vi "niDTS Comm String Initialize.vi"(0 "Session Name ()":string, 5 "Plugin Path":path, 7 "Logger":T2, 11 "error in (no error)":errorcluster) -> (4 "Comm String Handle":T1, 15 "error out":errorcluster)   [LabVIEW 2015, in "niDTS CommLib.lvlib"]
uses:
  niDTS CommLib.lvlib
  Framework/Logger/Includes/niDTS Logger INC Handle.ctl
  Framework/Logger/Objects/BASE_class/niDTS Logger.lvclass
  Includes/niDTS Comm String INC Handle.ctl
  Objects/String_class/niDTS Comm String.lvclass
  Framework/Session/Objects/BASE_class/niDTS Session.lvclass
  Framework/niDTS Framework.lvlib
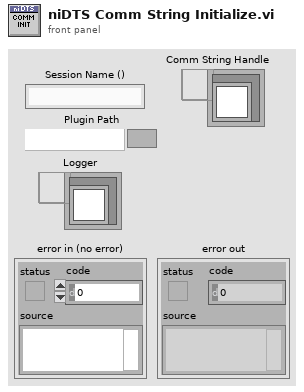
[diagram p1: front panel]
types:
  T1 = typedef "niDTS CommLib.lvlib/niDTS Comm String INC Handle.ctl" = refnum<data-value>
  T2 = typedef "niDTS Framework.lvlib/niDTS Logger INC Handle.ctl" = refnum<data-value>
  T3 = typedef "niDTS Framework.lvlib/niDTS Session INC Handle.ctl" = refnum<data-value>
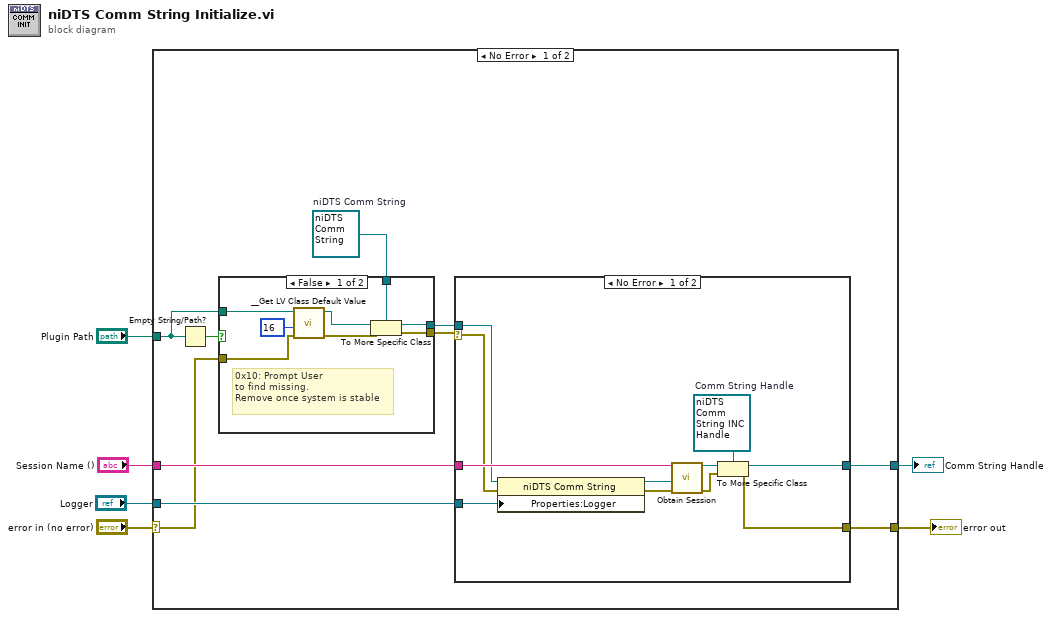
[diagram p0: block diagram]
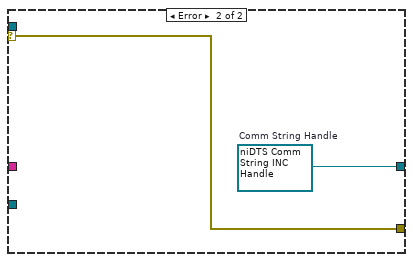
[diagram p2: hidden frame]
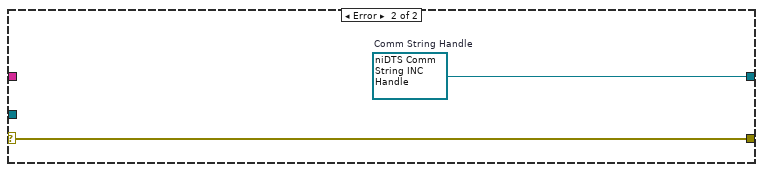
[diagram p4: hidden frame]
diagram:
  n1 = case shown="No Error" "error in (no error)" {
    selector: "error in (no error)" -> [w10 w41]
    tunnel: "Session Name ()" -> [w16 _]
    tunnel: [w15 w41] -> w5
    tunnel: "Logger" -> [w14 _]
    tunnel: "Plugin Path" -> [w11 _]
    tunnel: [w7 w40] -> w1
    frame No Error {
      w12 = refnum<class "niDTS Comm String.lvclass"> refnum  # niDTS Comm String
      n2 = Empty String/Path?(string/path=w11) -> (empty?=w13:bool)
      n3 = case shown="False" w13 {
        tunnel: [w32 w39] -> w8
        tunnel: w11 -> [w37 _]
        tunnel: w10 -> [w35 w38]
        tunnel: w12 -> [w33 w39]
        tunnel: [w31 w38] -> w9
        frame False {
          # "0x10: Prompt User\nto find missing. \nRemove once system is stable"
          n4 = call "__Get LV Class Default Value.vi"("error in (no error)"=w35, "options"=u32 16, "class path"=w37) -> ("error out"=w34:errorcluster, "object"=w30:refnum<class>)  [unwired: 7 in]
          n5 = To More Specific Class(target class=w33, reference=w30, error in=w34) -> (specific class reference=w32:refnum<class "niDTS Comm String.lvclass">, error out=w31:errorcluster)
        }
        frame True {
        }
      }
      n6 = case shown="No Error" w9 {
        selector: w9 -> [w17 w29]
        tunnel: w16 -> [w27 _]
        tunnel: [w25 w29] -> w15
        tunnel: [w22 w28] -> w7
        tunnel: w14 -> [w19 _]
        tunnel: w8 -> [w18 _]
        frame No Error {
          w24 = T1 refnum  # Comm String Handle
          n7 = property class="niDTS Comm String"(reference=w18, error in=w17, "Properties:Logger"=w19) -> (reference out=w21:refnum<class "niDTS Comm String.lvclass">, error out=w20:errorcluster)
          n8 = call "Obtain Session.vi"("Session Name ()"=w27, "OBJ - Session"=w21, "error in (no error)"=w20) -> ("Session Handle"=w23:T3, "error out"=w26:errorcluster)  [unwired: 10 in, 1 out]
          n9 = To More Specific Class(target class=w24, reference=w23, error in=w26) -> (specific class reference=w22:T1, error out=w25:errorcluster)
        }
        frame Error {
          w28 = T1 refnum  # Comm String Handle
        }
      }
    }
    frame Error {
      w40 = T1 refnum  # Comm String Handle
    }
  }
  "error out" <- w5
  "Comm String Handle" <- w1
